vi "Autotuning PID Offline.vi"() -> ()   [LabVIEW 2023]
doc: "This example demonstrates how to use the PID Design function to obtain PID parameters based on measured process."
uses:
  <vilib>/addons/control/pid/pid.llb/PID Advanced (DBL).vi
  <vilib>/addons/control/pid/autopid.llb/PID Autotuning Design (Ziegler-Nichols).vi
  <vilib>/addons/control/pid/autopid.llb/PID Autotuning Design (Cohen-Coon).vi
  <vilib>/addons/control/pid/autopid.llb/PID Autotuning Design (Chien-Hrones-Reswick).vi
  <vilib>/addons/control/pid/autopid.llb/PID Autotuning Design (Internal Model Control).vi
  <vilib>/addons/control/pid/NI_PID_autopid.lvlib
  <vilib>/addons/control/pid/NI_PID_pid.lvlib
  <vilib>/ptbypt/NI_PtbyPt.lvlib
panel:
  in  "Excitation":dbl=0.5 format="%.2f"
  in  "Type of controller":u16(ring)=2 items=["P", "PI", "PID"]
  in  "Control":T1(tab)
  in  "Ziegler-Nichols speed":u16(ring) items=["Fast", "Normal", "Slow"]
  in  "Tuning specifications":u16(ring) items=["Regulator - 0 %", "Regulator -  20%", "Servo - 0%", "Servo - 20%"]
  in  "Multiplicative factor":dbl(slide)=1.0 scale=0.01..100.0
  in  "Tab Control":T2(tab)
  in  "Instructions":string="Overview: This example demonstrates how to use the PID Autotuning Design to obtain PID parameters based on setpoint and process variable collected in another loop.\nInstructions:\n1. Run the VI and wait until the process variable (PV) reaches near setpoint (SP).\n2.  In the PID Autotuning Design section, select the type of algorithm, type of controller and excitation amplitude for the 'open loop step response'. Then, click Autotune to start the process. Select the Identified Plant Parameter tab and see the results from the identification.\n3.  When the tuned PID gains do not change anymore, the identification is done and you have the option to accept by clicking Accept gain, which will transfer the new gain to PID Gains.\n4. Click the Autotune button again to go back to the automatic control state. You can try different options and repeat this process.\n5. Click Stop to stop the VI.\n"
  out "Identified Plant Parameters":T3={"Plant Gain (K)"=1.7609511324977591, "Time Constant (T)"=1.9621978490901302, "Dead Time (L)"=0.22467425343567116}
  out "Control Output":dbl[](graph)
  out "Measurement":dbl[](graph)
  out "Stimulus operating point":dbl=20.314221540357543
  out "Response operating point":dbl=51.08345461694337
  in  "Automatic":bool=TRUE
  in  "Reinitialize":bool
  out "MV":dbl(graph)=20.39115328927357
  in  "Accept gain":bool
  out "Tuned PID gains":T4={"proportional gain (Kc)"=1.9838195929127882, "integral time (Ti, min)"=0.01995856284686879, "derivative time (Td, min)"=0.0} {"derivative time (Td, min)" format="%#.6g"; "integral time (Ti, min)" format="%#.6g"; "proportional gain (Kc)" format="%#.6g"}
  in  "Autotune":bool
  in  "SP:":dbl(slide)=50.98039215686275 min=0.0 max=0.0 scale=0.0..100.0
  in  "MV:":dbl(slide)=20.39115328927357 scale=-100.0..100.0
  out "PV:":dbl(slide)=50.98160323470328 scale=0.0..100.0
  in  "PID Gains":T4={"proportional gain (Kc)"=2.5, "integral time (Ti, min)"=0.02, "derivative time (Td, min)"=0.0} {"derivative time (Td, min)" format="%#.6g"; "integral time (Ti, min)" format="%#.6g"; "proportional gain (Kc)" format="%#.6g"}
  in  "Sampling Time dt (s)":dbl=0.05 min=0.001 step=0.01 format="%#.3p"
  in  "Stop":bool
  out "SP and PV":cluster{"initial PV":dbl, "SP1:":dbl}(graph)={"initial PV"=50.98160323470328, "SP1:"=50.98039215686275}
  # "Proportional-Integral-Derivative (PID) Controller"
  # "PID Autotuning Design"
  # "No additional parameters"
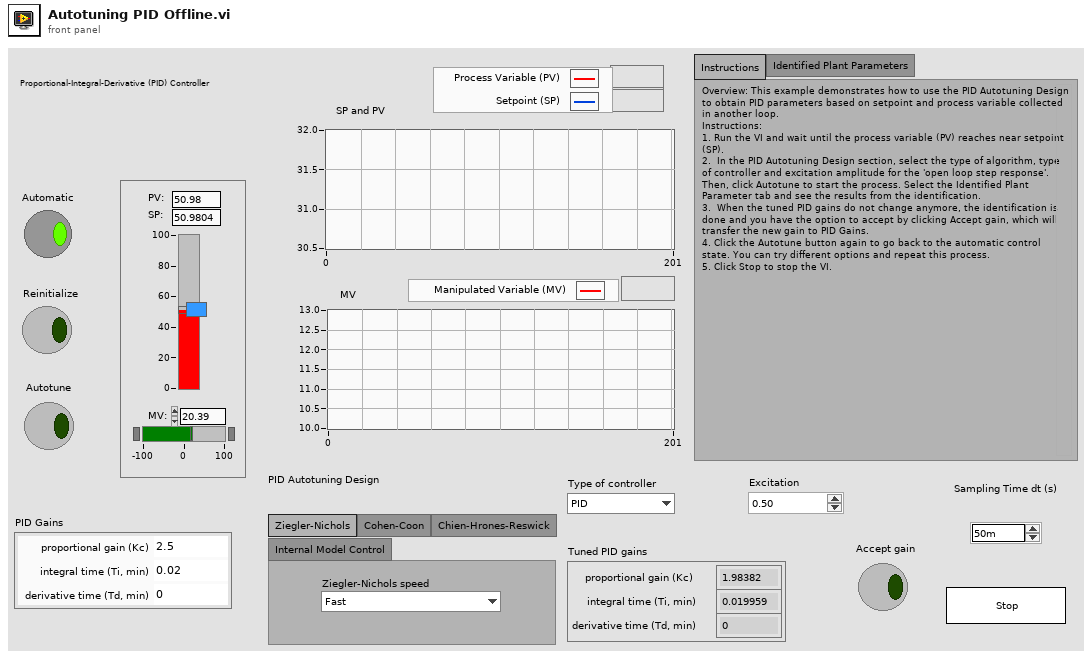
[diagram p1: front panel]
types:
  T1 = enum32{"Ziegler-Nichols", "Cohen-Coon", "Chien-Hrones-Reswick", "Internal Model Control"}
  T2 = enum32{"Instructions", "Identified Plant Parameters"}
  T3 = cluster{"Plant Gain (K)":dbl, "Time Constant (T)":dbl, "Dead Time (L)":dbl}
  T4 = cluster{"proportional gain (Kc)":dbl, "integral time (Ti, min)":dbl, "derivative time (Td, min)":dbl}
  T5 = cluster{"static gain":dbl, "lag (s)":dbl, "deadtime (s)":dbl, "load":dbl, "deadband":dbl, "sensor noise":dbl, "initial PV":dbl, "plant noise":dbl}
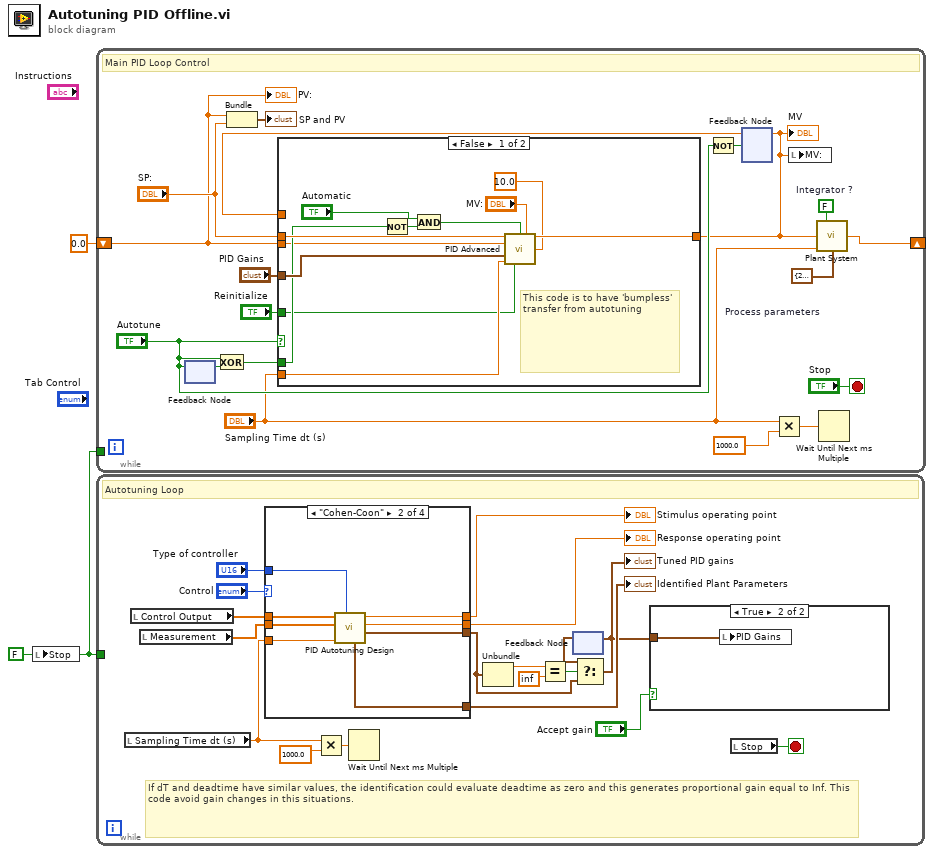
[diagram p0: block diagram]
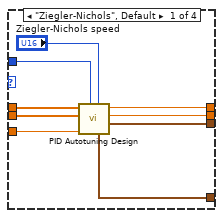
[diagram p2: hidden frame]
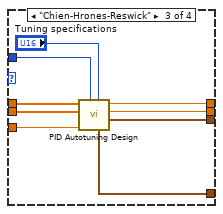
[diagram p3: hidden frame]
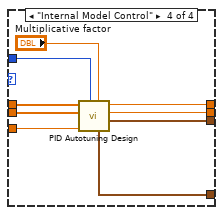
[diagram p4: hidden frame]
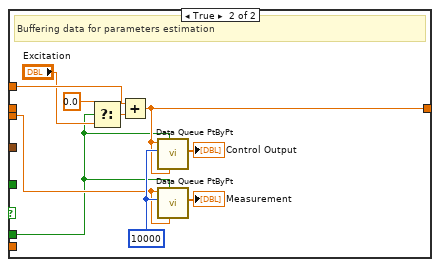
[diagram p6: hidden frame]
diagram:
  w1 = FALSE ("Stop")
  n1 = local write "Stop"(w1) -> ()
  n2 = while {
    shift-left: 0.0 ("Plant Output") -> [w13]
    shift-right: [w8] -> _
    tunnel: w1 -> [_]
    stop <- "Stop" stop-if-true
    w7 = T5 {"static gain"=2.5, "lag (s)"=2.5, "deadtime (s)"=0.01, "load"=0.0, "deadband"=0.0, "sensor noise"=0.0, "initial PV"=30.0, "plant noise"=0.0}  # Process parameters
    w9 = FALSE  # Integrator ?
    # "Main PID Loop Control"
    n3 = feedback #1() -> (w15:bool)  [unwired: 1 in]
    n4 = feedback-in #1("Autotune") -> ()
    n5 = Exclusive Or(1:w15, 2:"Autotune") -> (0:w14:bool)
    n6 = Bundle("Plant Output"=w13, "SP:"="SP:") -> (→"SP and PV":cluster{"Plant Output":dbl, "SP:":dbl})  [unwired: 1 in]
    n7 = Not(x="Autotune") -> (.not. x?=w10:bool)
    n8 = feedback #2() -> (w12:dbl)  [unwired: 1 in]
    n9 = case shown="False" "Autotune" {
      tunnel: "Sampling Time dt (s)" -> [w32 _]
      tunnel: [w30 w35] -> w6
      tunnel: w13 -> [w27 w34]
      tunnel: "SP:" -> [w29 _]
      tunnel: "PID Gains" -> [w31 _]
      tunnel: "Reinitialize" -> [w25 _]
      tunnel: w14 -> [w28 w33]
      tunnel: w12 -> [_ w39]
      frame False {
        # "This code is to have 'bumpless' transfer from autotuning"
        n10 = Not(x=w28) -> (.not. x?=w24:bool)
        n11 = And(x="Automatic", y=w24) -> (x .and. y?=w26:bool)
        n12 = call-poly <vilib>:"PID Advanced.vi"("setpoint"=w29, "auto? (T)"=w26, "manual control"="MV:", "process variable"=w27, "alpha"=10.0, "PID gains"=w31, "dt (s)"=w32, "reinitialize? (F)"=w25) -> ("output"=w30:dbl)  [unwired: 6 in, 1 out]
      }
      frame True {
        w42 = 10000 ("sample length")
        # "Buffering data for parameters estimation"
        n13 = Select(t=0.0, s=w33, f="Excitation") -> (s? t:f=w40:dbl)
        n14 = Add(x=w39, y=w40) -> (x+y=w35:dbl)
        n15 = call <vilib>:"Data Queue PtByPt.vi"("initial queue element"=w35, "initialize"=w33, "sample length"=w42, "input data point"=w35) -> ("Current Queue"=→"Control Output":dbl[])  [unwired: 3 in, 4 out]
        n16 = call <vilib>:"Data Queue PtByPt.vi"("initial queue element"=w34, "initialize"=w33, "sample length"=w42, "input data point"=w34) -> ("Current Queue"=→"Measurement":dbl[])  [unwired: 3 in, 4 out]
      }
    }
    "MV" <- w6
    n17 = feedback-in #2(w6, w10) -> ()
    n18 = Multiply(x="Sampling Time dt (s)", y=1000.0) -> (x*y=w4:dbl)
    n19 = local write "MV:"(w6) -> ()
    n20 = call "Plant System.vi"("Integrator ?"=w9, "Plant Input"=w6, "dt (s)"="Sampling Time dt (s)", "process parameters"=w7) -> ("Plant Output"=w8:dbl)  [unwired: 11 in]
    n21 = Wait Until Next ms Multiple(millisecond multiple=w4) -> ()  [unwired: 1 out]
    "PV:" <- w13
  }
  n22 = while {
    tunnel: w1 -> [_]
    stop <- w55 stop-if-true
    # "If dT and deadtime have similar values, the identification could evaluate deadtime as zero and this generates proportional gain equal to Inf. This code avoid gain changes in this situations."
    # "Autotuning Loop"
    n23 = local read "Sampling Time dt (s)"() -> (w56:dbl)
    n24 = local read "Control Output"() -> (w60:dbl[])
    n25 = local read "Measurement"() -> (w59:dbl[])
    n26 = case shown="\"Cohen-Coon\"" "Control" {
      tunnel: w60 -> [w69 w77 w86 w95]
      tunnel: w59 -> [w68 w76 w85 w94]
      tunnel: [w67 w75 w84 w93] -> w58
      tunnel: [w66 w74 w83 w92] -> w57
      tunnel: w56 -> [w65 w73 w82 w91]
      tunnel: [w64 w72 w81 w90] -> w53
      tunnel: [w63 w71 w80 w89] -> w44
      tunnel: "Type of controller" -> [w62 w70 w79 w88]
      frame "Ziegler-Nichols", Default {
        n27 = call-poly <vilib>:"PID Autotuning Design.vi"("Ziegler-Nichols Speed"="Ziegler-Nichols speed", "Type of Controller"=w62, "dt (s)"=w65, "Response signal"=w68, "Stimulus signal"=w69) -> ("PID gains"=w63:T4, "response operating point"=w66:dbl, "stimulus operating point"=w67:dbl, "Plant Parameters"=w64:T3)  [unwired: 3 in]
      }
      frame "Cohen-Coon" {
        n28 = call-poly <vilib>:"PID Autotuning Design.vi"("Type of Controller"=w70, "dt (s)"=w73, "Response signal"=w76, "Stimulus signal"=w77) -> ("PID gains"=w71:T4, "response offset"=w74:dbl, "stimulus offset"=w75:dbl, "Plant Parameters"=w72:T3)  [unwired: 4 in]
      }
      frame "Chien-Hrones-Reswick" {
        n29 = call-poly <vilib>:"PID Autotuning Design.vi"("Tuning specifications"="Tuning specifications", "Type of Controller"=w79, "dt (s)"=w82, "Response signal"=w85, "Stimulus signal"=w86) -> ("PID gains"=w80:T4, "response offset"=w83:dbl, "stimulus offset"=w84:dbl, "Plant Parameters"=w81:T3)  [unwired: 3 in]
      }
      frame "Internal Model Control" {
        n30 = call-poly <vilib>:"PID Autotuning Design.vi"("Desired Time Constant (tau_c)"="Multiplicative factor", "Type of Controller"=w88, "dt (s)"=w91, "Response signal"=w94, "Stimulus signal"=w95) -> ("PID gains"=w89:T4, "response offset"=w92:dbl, "stimulus offset"=w93:dbl, "Plant Parameters"=w90:T3)  [unwired: 3 in]
      }
    }
    "Stimulus operating point" <- w58
    "Response operating point" <- w57
    "Identified Plant Parameters" <- w53
    n31 = Multiply(x=w56, y=1000.0) -> (x*y=w52:dbl)
    n32 = Wait Until Next ms Multiple(millisecond multiple=w52) -> ()  [unwired: 1 out]
    n33 = Unbundle(w44) -> ("proportional gain (Kc)"=w47:dbl)  [unwired: 2 out]
    n34 = Equal?(x=w47, y=inf) -> (x = y?=w46:bool)
    n35 = feedback #3() -> (w45:T4)  [unwired: 1 in]
    n36 = Select(t=w45, s=w46, f=w44) -> (s? t:f=w43:T4)
    "Tuned PID gains" <- w43
    n37 = feedback-in #3(w43) -> ()
    n38 = case shown="True" "Accept gain" {
      tunnel: w43 -> [_ w96]
      frame False {
      }
      frame True {
        n39 = local write "PID Gains"(w96) -> ()
      }
    }
    n40 = local read "Stop"() -> (w55:bool)
  }
